vi "load_class.vi"(8 "error in (no error)":errorcluster, 11 "builder_class in":path) -> (0 "error out":errorcluster, 1 "name":string, 2 "lv_builder":refnum<class "lv-builder.lvclass">, 3 "builder_class out":path)   [LabVIEW 2015, in "lv-builder.lvlib"]
uses:
  lv-builder.lvlib
  lv-builder.lvclass
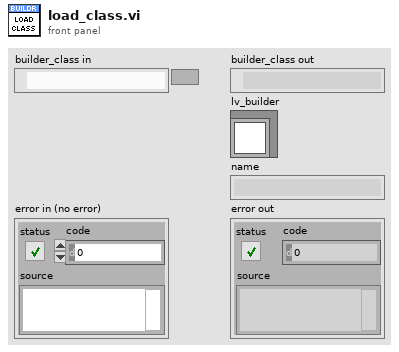
[diagram p1: front panel]
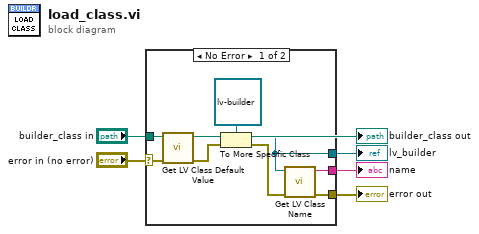
[diagram p0: block diagram]
diagram:
  n1 = case shown="No Error" "error in (no error)" {
    selector: "error in (no error)" -> [w11 w15]
    tunnel: [w9 _] -> w5
    tunnel: [w7 w15] -> w4
    tunnel: "builder_class in" -> [w12 _]
    tunnel: [w6 _] -> w1
    frame No Error {
      n2 = call <vilib>:"Get LV Class Default Value.vi"("error in (no error)"=w11, "class path"=w12) -> ("error out"=w13:errorcluster, "object"=w14:refnum<class>)  [unwired: 8 in]
      n3 = To More Specific Class(target class=refnum<class "lv-builder.lvclass"> refnum ("lv-build.lvlib:lv-build.lvclass"), reference=w14, error in=w13) -> (specific class reference=w9:refnum<class "lv-builder.lvclass">, error out=w8:errorcluster)
      n4 = call <vilib>:"Get LV Class Name.vi"("error in (no error)"=w8, "object"=w9) -> ("error out"=w7:errorcluster, "class name"=w6:string)  [unwired: 8 in]
    }
    frame Error {
    }
  }
  "error out" <- w4
  "lv_builder" <- w5
  "name" <- w1
  "builder_class out" <- "builder_class in"
